vi "io-find-by-type.vi"(9 "Mode(Any)":T1, 10 "Type":T4=enum."DI", 11 "IOConfigs in":T2[](array[typedef]) {"calibration"."Y" format="%#.3f"; "calibration"."X" format="%#.3f"; "ADDR" format="%04d"}) -> (3 "Search Results":T2[](array[typedef]) {"calibration"."Y" format="%#.3f"; "calibration"."X" format="%#.3f"; "ADDR" format="%04d"})   [LabVIEW 2024]
uses:
  controls/IONode.ctl
  controls/type.address.ctl
  controls/enum.io.type.ctl
  controls/enum.io.mode.ctl
  controls/typeXyPoint.ctl
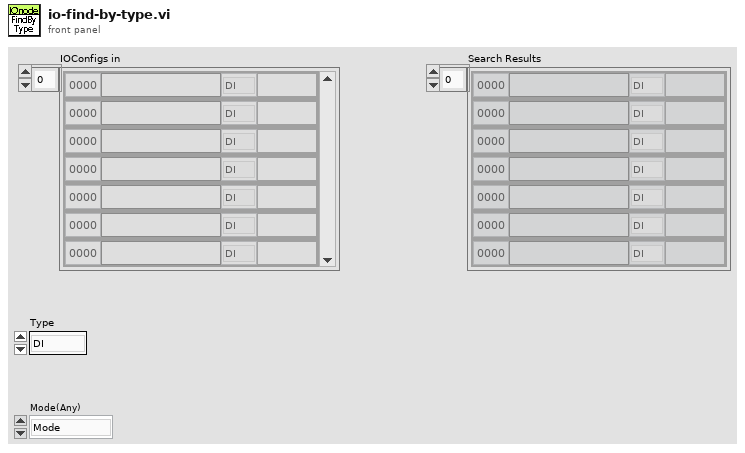
[diagram p1: front panel]
types:
  T1 = typedef "enum.io.mode.ctl" = enum16{"Mode", "RIO", "SIM"}
  T2 = typedef "IONode.ctl" = cluster{"ADDR":T3, "Label":string, "Type":T4, "Mode":T1, "Value":string, "Tags":string, "calibration":T5[]}
  T3 = typedef "type.address.ctl" = u16
  T4 = typedef "enum.io.type.ctl" = enum16{"Type", "DI", "DO", "AI", "AO", "VL", "BUF"}
  T5 = typedef "typeXyPoint.ctl" = cluster{"X":dbl, "Y":dbl}
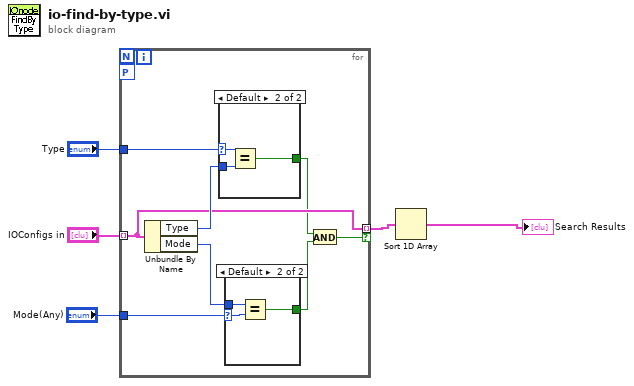
[diagram p0: block diagram]
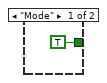
[diagram p2: hidden frame]
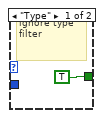
[diagram p3: hidden frame]
diagram:
  n1 = for {
    tunnel: "IOConfigs in" -> [w12] mode=indexing
    tunnel: "Type" -> [w7]
    tunnel: [w12] -> w2 mode=indexing if=w9
    tunnel: "Mode(Any)" -> [w6]
    workers-P: _ -> [_]
    n2 = Unbundle By Name(w12) -> ("Type"=w13:T4, "Mode"=w10:T1)
    n3 = case shown="Default" w7 {
      selector: w7 -> [_ w19]
      tunnel: w13 -> [_ w21]
      tunnel: [TRUE w20] -> w11
      frame "Type" {
        # "ignore type filter"
      }
      frame Default {
        n4 = Equal?(x=w19, y=w21) -> (x = y?=w20:bool)
      }
    }
    n5 = case shown="Default" w6 {
      selector: w6 -> [_ w15]
      tunnel: w10 -> [_ w17]
      tunnel: [TRUE w16] -> w8
      frame "Mode" {
      }
      frame Default {
        n6 = Equal?(x=w17, y=w15) -> (x = y?=w16:bool)
      }
    }
    n7 = And(x=w11, y=w8) -> (x .and. y?=w9:bool)
  }
  n8 = Sort 1D Array(array=w2) -> (sorted array=→"Search Results":T2[])
